vi "Loopback.vi"() -> ()   [LabVIEW 2020]
uses:
  <vilib>/eio/EIONode/EIONode.xnode
  <vilib>/rvi/eio/common/nirviEmuTemplateMethod_errors.vi
panel:
  out "Current Counter":u8
  in  "Use Counter?":bool=TRUE
  in  "Connector0/DIOPORT3":u8
  in  "Connector0/DIOPORT0":u8
  out "Connector0/DIOPORT2":u8 format="%.0b"
  out "Connector0/DIOPORT1":u8 format="%.0b"
  in  "Wait (mSec)":u32 caption="Count(mSec)"
  in  "Reset Counter?":bool
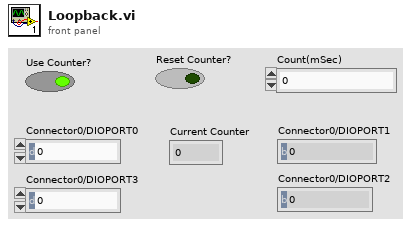
[diagram p1: front panel]
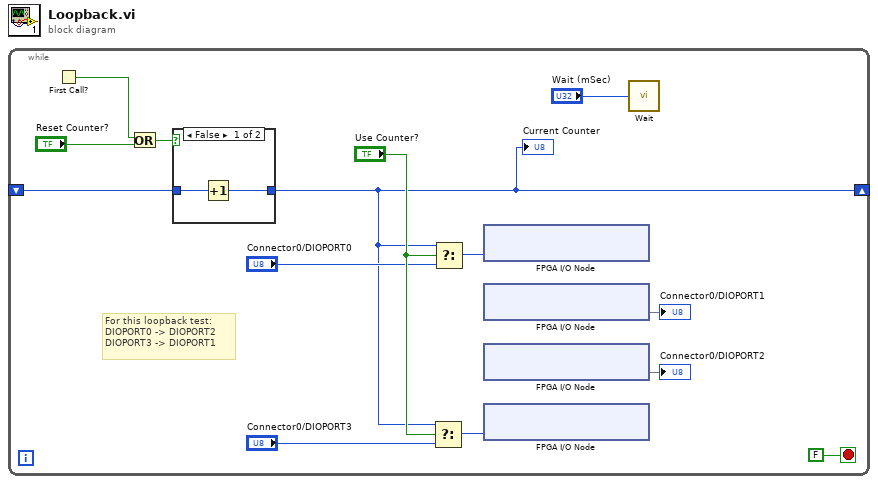
[diagram p0: block diagram]
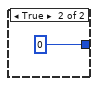
[diagram p2: hidden frame]
diagram:
  n1 = while {
    shift-right: [w1] -> _
    shift-left: _ -> [w13]
    stop <- FALSE stop-if-true
    # "For this loopback test:\nDIOPORT0 -> DIOPORT2\nDIOPORT3 -> DIOPORT1"
    n2 = First Call?() -> (First Call?: T/F=w11:bool)
    n3 = Or(x=w11, y="Reset Counter?") -> (x .or. y?=w10:bool)
    n4 = case shown="False" w10 {
      tunnel: [w15 u8 0] -> w1
      tunnel: w13 -> [w16 _]
      frame False {
        n5 = Increment(x=w16) -> (x+1=w15:u8)
      }
      frame True {
      }
    }
    "Current Counter" <- w1
    n6 = Select(t=w1, s="Use Counter?", f="Connector0/DIOPORT3") -> (s? t:f=w5:u8)
    n7 = Select(t=w1, s="Use Counter?", f="Connector0/DIOPORT0") -> (s? t:f=w6:u8)
    n8 = xnode "FPGA I/O Node"("Connector0/DIOPORT0"=w6) -> ()  [unwired: 1 in, 1 out]
    n9 = xnode "FPGA I/O Node"() -> ("Connector0/DIOPORT1"=→"Connector0/DIOPORT1")  [unwired: 1 in, 1 out]
    n10 = xnode "FPGA I/O Node"() -> ("Connector0/DIOPORT2"=→"Connector0/DIOPORT2")  [unwired: 1 in, 1 out]
    n11 = xnode "FPGA I/O Node"("Connector0/DIOPORT3"=w5) -> ()  [unwired: 1 in, 1 out]
    n12 = call "Wait"("Count(mSec)"="Wait (mSec)") -> ()  [unwired: 1 out]
  }
